vi "Set Segmenting Specification (Footprint).vi"(5 "Segment File on Trigger (T)":bool=TRUE, 7 "Max Instances (-1: Infinite)":i32=-1, 8 "error in (no error)":errorcluster, 9 "Size Check Period (1000 ms)":u32=1000, 10 "Size":u64, 11 "Data Logging Specification Ref in":T1) -> (0 "error out":errorcluster, 3 "Data Logging Specification Ref out":T1)   [LabVIEW 2020, in "NI_VS Data Logging API.lvlib"]
doc: "Specifies how to segment the log files created during the data logging session. You can segment log files according to time or size limits, or when a start trigger occurs. When the segmenting condition is met, this VI saves and closes the current log file and continues logging data in a new file.\n\nSelect the Default instance of this VI if you do not want to segment log files based on time or size, but do want the option to segment on a start trigger.\n\nYou must manually select the polymorphic instance to use."
uses:
  <vilib>/NI VeriStand/Execution/DataLogging/NI_VS Data Logging API.lvlib
  <vilib>/NI VeriStand/Execution/DataLogging/DataLoggingSpecification Ref.ctl
  NationalInstruments.VeriStand.ClientAPI
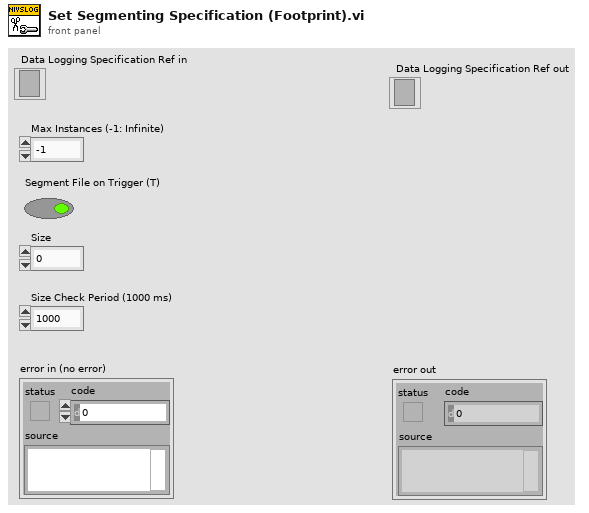
[diagram p1: front panel]
types:
  T1 = typedef "NI_VS Data Logging API.lvlib/DataLoggingSpecification Ref.ctl" = refnum<k24>
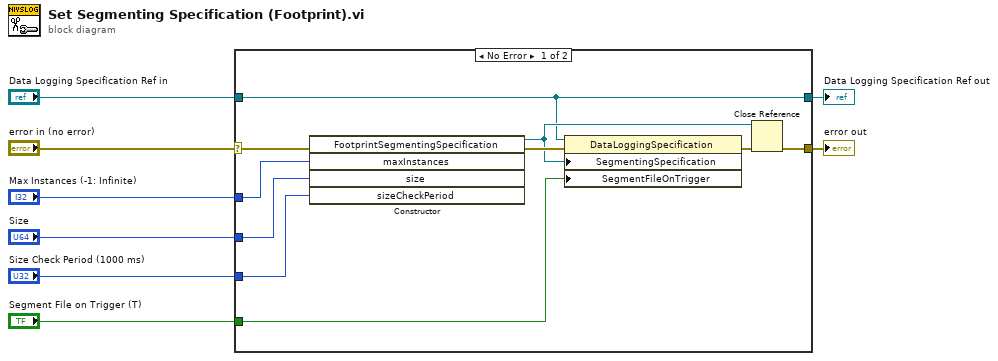
[diagram p0: block diagram]
diagram:
  n1 = case shown="No Error" "error in (no error)" {
    selector: "error in (no error)" -> [w18 w20]
    tunnel: [w14 w20] -> w7
    tunnel: [w12 w19] -> w6
    tunnel: "Data Logging Specification Ref in" -> [w12 w19]
    tunnel: "Max Instances (-1: Infinite)" -> [w17 _]
    tunnel: "Segment File on Trigger (T)" -> [w11 _]
    tunnel: "Size" -> [w10 _]
    tunnel: "Size Check Period (1000 ms)" -> [w9 _]
    frame No Error {
      n2 = constructor class="FootprintSegmentingSpecificatio"(error in=w18, "maxInstances"=w17, "size"=w10, "sizeCheckPeriod"=w9) -> (reference out=w13:refnum<k24>, error out=w16:errorcluster)  [unwired: 2 in, 4 out]
      n3 = property class="DataLoggingSpecification"(reference=w12, error in=w16, "SegmentingSpecification"=w13, "SegmentFileOnTrigger"=w11) -> (error out=w15:errorcluster)  [unwired: 1 out]
      n4 = Close Reference(reference=w13, error in (no error)=w15) -> (error out=w14:errorcluster)
    }
    frame Error {
    }
  }
  "error out" <- w7
  "Data Logging Specification Ref out" <- w6
